vi "Choreo_TrajectoryDifferential_GetFinalPose.vi"(9 "mirrorForRedAlliance":bool, 11 "ChoreoTrajectoryDifferential":T4) -> (1 "Exists":bool, 3 "FinalPose":T1={"TRANSLATION"={"X"=0.0, "Y"=0.0}, "ROTATION"={"VALUE"=0.0, "COS"=1.0, "SIN"=0.0}} {"ROTATION"."SIN" format="%13.4f"; "ROTATION"."COS" format="%13.4f"; "ROTATION"."VALUE" format="%13.4f"; "TRANSLATION"."Y" format="%14.3f"; "TRANSLATION"."X" format="%14.3f"})   [LabVIEW 2019, in "ChoreoLib.lvlib"]
doc: "Returns the final pose in the trajectory.\n \nThis function will return empty and Exists will be false.\n \nInputs: \n -- ChoreoTrajectorySwerve - cluster - data cluster for this trajectory \n -- mirrorForRedAlliance - boolean - whether or not to return the sample as mirrored across the field\n\nOutputs: \n -- FinalPose - pose2d - The final pose in the trajectory.\n -- exists - boolean - the sample exits."
uses:
  ChoreoLib.lvlib
  TypeDef/ChoreoTrajectoryDifferential.ctl
  TypeDef/ChoreoDifferentialSample.ctl
  TypeDef/ChoreoEventMarker.ctl
  <vilib>/Rock Robotics/WPI/ThirdParty/JAS_Junk/TrajLib/TypeDef/POSE2D.ctl
  <vilib>/Rock Robotics/WPI/ThirdParty/JAS_Junk/TrajLib/TypeDef/TRANSLATION2D.ctl
  <vilib>/Rock Robotics/WPI/ThirdParty/JAS_Junk/TrajLib/TypeDef/ROTATION2D.ctl
  <vilib>/Rock Robotics/WPI/ThirdParty/JAS_Junk/TrajLib/Pose2d_New.vi
  <vilib>/Rock Robotics/WPI/ThirdParty/JAS_Junk/TrajLib/Rotation2d_CreateAngle.vi
  <vilib>/Rock Robotics/WPI/ThirdParty/JAS_Junk/TrajLib/Translation2d_Create.vi
  <vilib>/Rock Robotics/WPI/ThirdParty/JAS_Junk/TrajLib/Trajectory_Library.lvlib
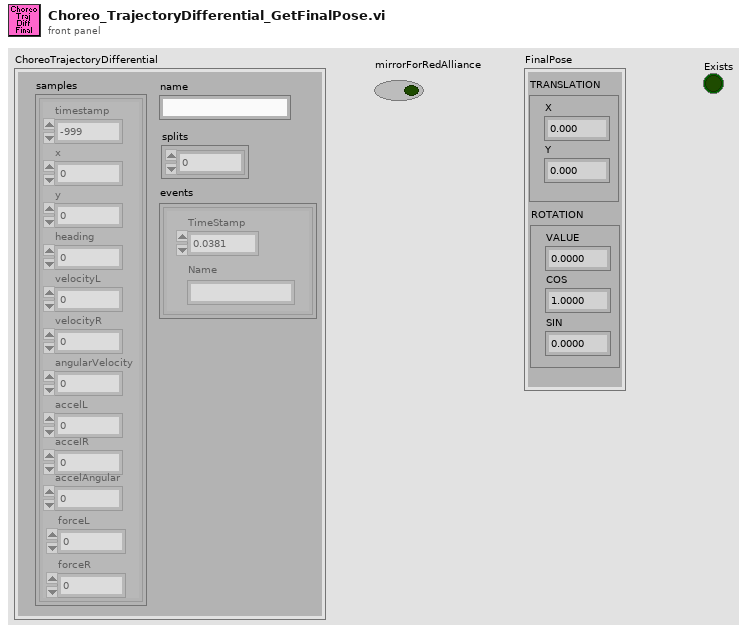
[diagram p1: front panel]
types:
  T1 = typedef "Trajectory_Library.lvlib/POSE2D.ctl" = cluster{"TRANSLATION":T2, "ROTATION":T3}
  T2 = typedef "Trajectory_Library.lvlib/TRANSLATION2D.ctl" = cluster{"X":dbl, "Y":dbl}
  T3 = typedef "Trajectory_Library.lvlib/ROTATION2D.ctl" = cluster{"VALUE":dbl, "COS":dbl, "SIN":dbl}
  T4 = typedef "ChoreoLib.lvlib/ChoreoTrajectoryDifferential.ctl" = cluster{"name":string, "samples":T5[], "splits":i32[], "events":T6[]}
  T5 = typedef "ChoreoLib.lvlib/ChoreoDifferentialSample.ctl" = cluster{"timestamp":dbl, "x":dbl, "y":dbl, "heading":dbl, "velocityL":dbl, "velocityR":dbl, "angularVelocity":dbl, "accelL":dbl, "accelR":dbl, "accelAngular":dbl, "forceL":dbl, "forceR":dbl}
  T6 = typedef "ChoreoLib.lvlib/ChoreoEventMarker.ctl" = cluster{"TimeStamp":dbl, "Name":string}
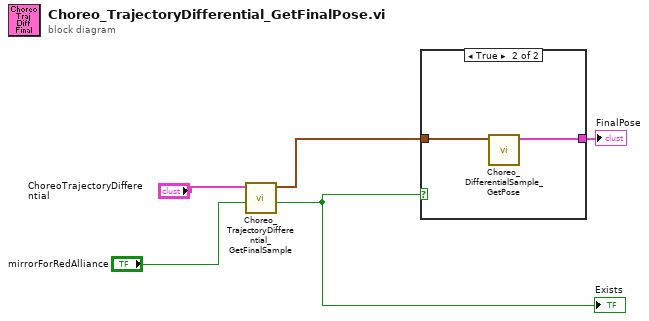
[diagram p0: block diagram]
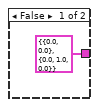
[diagram p2: hidden frame]
diagram:
  n1 = call "Choreo_TrajectoryDifferential_GetFinalSample.vi"("mirrorForRedAlliance"="mirrorForRedAlliance", "ChoreoTrajectoryDifferential"="ChoreoTrajectoryDifferential") -> ("Exists"=w3:bool, "sample"=w2:T5)  [unwired: 8 in]
  "Exists" <- w3
  n2 = case shown="True" w3 {
    tunnel: w2 -> [_ w8]
    tunnel: [T1 {"TRANSLATION"={"X"=0.0, "Y"=0.0}, "ROTATION"={"VALUE"=0.0, "COS"=1.0, "SIN"=0.0}} ("Pose") w7] -> w1
    frame False {
    }
    frame True {
      n3 = call "Choreo_DifferentialSample_GetPose.vi"("ChoreoDifferentialSample"=w8) -> ("Pose"=w7:T1)  [unwired: 10 in]
    }
  }
  "FinalPose" <- w1
